vi "OpenCVcircleFinder.vi"() -> ()   [LabVIEW 2019]
panel:
  out "return value":u16[](array[numeric])
  out "error out":errorcluster
  in  "Function Name":string="circleDetectorPCB"
  in  "Input File":string="C:\\\\Users\\\\TTUHEP\\\\Pictures\\\\LaserHoleColor.png"
  in  "Python Path":path=path "C:/Users/TTUHEP/Documents/LabVIEW/GantryPrograms/Utilities/circleDetector.py"
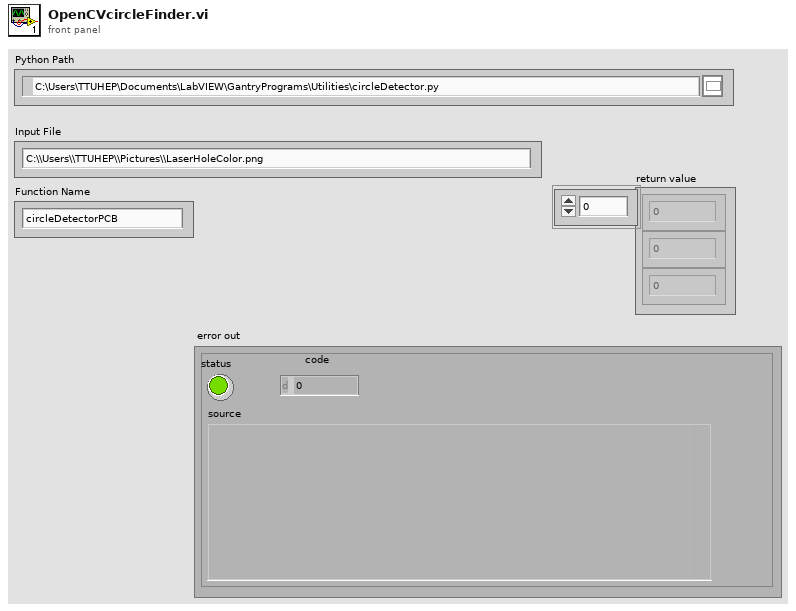
[diagram p1: front panel]
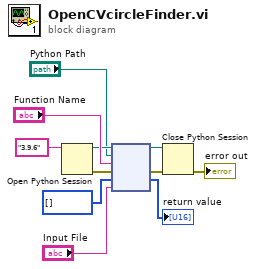
[diagram p0: block diagram]
diagram:
  n1 = Open Python Session(python version="3.9.6") -> (session out=w9:refnum<k35>, error out=w6:errorcluster)  [unwired: 2 in]
  n2 = node(w9, "Python Path", "Function Name", w6, u16[] [], "Input File") -> (w7:refnum<k35>, w5:errorcluster, →"return value":u16[])  [unwired: 1 in, 2 out]
  n3 = Close Python Session(session in=w7, error in=w5) -> (11:→"error out":errorcluster)
